vi "Convert EGU to V.vi"(0 "Sensors Info":T1(array[cluster])=[{"Sensor Name"="AI 0", "Sensor Info"={"Manufacturer"="", "Model"="", "Serial Number"=""}, "Last Cal Info"={"Last Calibration Date"=3153588337.646, "Calibrator"="", "Cal Duration"=0}, "Voltage Range"={"High Limit"=5.0, "Low Limit"=-5.0}, "EGU Range"={"High Limit"=-10000.0, "Low Limit"=10000.0}, "Units"="ue", "Calibration Type"=enum."Calibrate Analog", "EGU List"=[0.0, 10000.0, 20000.0], "Voltage List"=[0.0, 5.0, 7.0], "Coefficients"=[5.90433951730418e-12, -142.85714285714278, 428.5714285714284], "Order"=2, "Algorithm"=enum."SVD", "Max Error % of Full Scale"=0.0, "Max Mean Squared Error"=0.0, "Use Error %"=FALSE, "Use MSE"=FALSE, "Allow Manual Entry"=FALSE, "Max Stability Error"=2.0, "Max Error % of Reading"=0.0, "Use Error % of Reading"=FALSE}, {"Sensor Name"="AI 1", "Sensor Info"={"Manufacturer"="", "Model"="", "Serial Number"=""}, "Last Cal Info"={"Last Calibration Date"=3153957180.311, "Calibrator"="", "Cal Duration"=0}, "Voltage Range"={"High Limit"=5.0, "Low Limit"=-5.0}, "EGU Range"={"High Limit"=-10000.0, "Low Limit"=10000.0}, "Units"="ue", "Calibration Type"=enum."Calibrate Analog", "EGU List"=[0.0, 10000.0], "Voltage List"=[0.0, 5.0], "Coefficients"=[-0.0, 2000.0], "Order"=2, "Algorithm"=enum."SVD", "Max Error % of Full Scale"=0.0, "Max Mean Squared Error"=0.0, "Use Error %"=FALSE, "Use MSE"=FALSE, "Allow Manual Entry"=FALSE, "Max Stability Error"=2.0, "Max Error % of Reading"=0.0, "Use Error % of Reading"=FALSE}, {"Sensor Name"="AI 12", "Sensor Info"={"Manufacturer"="", "Model"="", "Serial Number"=""}, "Last Cal Info"={"Last Calibration Date"=3153952477.529, "Calibrator"="", "Cal Duration"=0}, "Voltage Range"={"High Limit"=0.0, "Low Limit"=10.0}, "EGU Range"={"High Limit"=0.0, "Low Limit"=10.0}, "Units"="Volts", "Calibration Type"=enum."Calibrate Analog", "EGU List"=[0.0, 10000.0], "Voltage List"=[0.0, 5.0], "Coefficients"=[-0.0, 2000.0], "Order"=2, "Algorithm"=enum."SVD", "Max Error % of Full Scale"=0.0, "Max Mean Squared Error"=0.0, "Use Error %"=FALSE, "Use MSE"=FALSE, "Allow Manual Entry"=FALSE, "Max Stability Error"=2.0, "Max Error % of Reading"=0.0, "Use Error % of Reading"=FALSE}, {"Sensor Name"="AI 13", "Sensor Info"={"Manufacturer"="", "Model"="", "Serial Number"=""}, "Last Cal Info"={"Last Calibration Date"=3153952479.4309998, "Calibrator"="", "Cal Duration"=0}, "Voltage Range"={"High Limit"=0.0, "Low Limit"=10.0}, "EGU Range"={"High Limit"=0.0, "Low Limit"=10.0}, "Units"="Volts", "Calibration Type"=enum."Calibrate Analog", "EGU List"=[0.0, 10000.0], "Voltage List"=[0.0, 5.0], "Coefficients"=[-0.0, 2000.0], "Order"=2, "Algorithm"=enum."SVD", "Max Error % of Full Scale"=0.0, "Max Mean Squared Error"=0.0, "Use Error %"=FALSE, "Use MSE"=FALSE, "Allow Manual Entry"=FALSE, "Max Stability Error"=2.0, "Max Error % of Reading"=0.0, "Use Error % of Reading"=FALSE}, {"Sensor Name"="AI 14", "Sensor Info"={"Manufacturer"="", "Model"="", "Serial Number"=""}, "Last Cal Info"={"Last Calibration Date"=3153952481.104, "Calibrator"="", "Cal Duration"=0}, "Voltage Range"={"High Limit"=0.0, "Low Limit"=10.0}, "EGU Range"={"High Limit"=0.0, "Low Limit"=10.0}, "Units"="Volts", "Calibration Type"=enum."Calibrate Analog", "EGU List"=[0.0, 10000.0], "Voltage List"=[0.0, 5.0], "Coefficients"=[-0.0, 2000.0], "Order"=2, "Algorithm"=enum."SVD", "Max Error % of Full Scale"=0.0, "Max Mean Squared Error"=0.0, "Use Error %"=FALSE, "Use MSE"=FALSE, "Allow Manual Entry"=FALSE, "Max Stability Error"=2.0, "Max Error % of Reading"=0.0, "Use Error % of Reading"=FALSE}, {"Sensor Name"="AI 15", "Sensor Info"={"Manufacturer"="", "Model"="", "Serial Number"=""}, "Last Cal Info"={"Last Calibration Date"=3153952482.786, "Calibrator"="", "Cal Duration"=0}, "Voltage Range"={"High Limit"=0.0, "Low Limit"=10.0}, "EGU Range"={"High Limit"=0.0, "Low Limit"=10.0}, "Units"="Volts", "Calibration Type"=enum."Calibrate Analog", "EGU List"=[0.0, 10000.0], "Voltage List"=[0.0, 5.0], "Coefficients"=[-0.0, 2000.0], "Order"=2, "Algorithm"=enum."SVD", "Max Error % of Full Scale"=0.0, "Max Mean Squared Error"=0.0, "Use Error %"=FALSE, "Use MSE"=FALSE, "Allow Manual Entry"=FALSE, "Max Stability Error"=2.0, "Max Error % of Reading"=0.0, "Use Error % of Reading"=FALSE}, {"Sensor Name"="AI 2", "Sensor Info"={"Manufacturer"="", "Model"="", "Serial Number"=""}, "Last Cal Info"={"Last Calibration Date"=3153588342.192, "Calibrator"="", "Cal Duration"=0}, "Voltage Range"={"High Limit"=5.0, "Low Limit"=-5.0}, "EGU Range"={"High Limit"=-10000.0, "Low Limit"=10000.0}, "Units"="ue", "Calibration Type"=enum."Calibrate Analog", "EGU List"=[0.0, 10000.0], "Voltage List"=[0.0, 5.0], "Coefficients"=[-0.0, 2000.0], "Order"=2, "Algorithm"=enum."SVD", "Max Error % of Full Scale"=0.0, "Max Mean Squared Error"=0.0, "Use Error %"=FALSE, "Use MSE"=FALSE, "Allow Manual Entry"=FALSE, "Max Stability Error"=2.0, "Max Error % of Reading"=0.0, "Use Error % of Reading"=FALSE}, {"Sensor Name"="AI 2", "Sensor Info"={"Manufacturer"="", "Model"="", "Serial Number"=""}, "Last Cal Info"={"Last Calibration Date"=3153844419.694, "Calibrator"="", "Cal Duration"=0}, "Voltage Range"={"High Limit"=0.0, "Low Limit"=10.0}, "EGU Range"={"High Limit"=0.0, "Low Limit"=10.0}, "Units"="Volts", "Calibration Type"=enum."Calibrate Analog", "EGU List"=[0.0, 10000.0], "Voltage List"=[0.0, 5.0], "Coefficients"=[-0.0, 2000.0], "Order"=2, "Algorithm"=enum."SVD", "Max Error % of Full Scale"=0.0, "Max Mean Squared Error"=0.0, "Use Error %"=FALSE, "Use MSE"=FALSE, "Allow Manual Entry"=FALSE, "Max Stability Error"=2.0, "Max Error % of Reading"=0.0, "Use Error % of Reading"=FALSE}, {"Sensor Name"="AI 3", "Sensor Info"={"Manufacturer"="", "Model"="", "Serial Number"=""}, "Last Cal Info"={"Last Calibration Date"=3153588411.1809998, "Calibrator"="", "Cal Duration"=0}, "Voltage Range"={"High Limit"=5.0, "Low Limit"=-5.0}, "EGU Range"={"High Limit"=-10000.0, "Low Limit"=10000.0}, "Units"="ue", "Calibration Type"=enum."Calibrate Analog", "EGU List"=[0.0, 10.0], "Voltage List"=[0.0, 5.0], "Coefficients"=[-0.0, 2.0], "Order"=2, "Algorithm"=enum."SVD", "Max Error % of Full Scale"=0.0, "Max Mean Squared Error"=0.0, "Use Error %"=FALSE, "Use MSE"=FALSE, "Allow Manual Entry"=FALSE, "Max Stability Error"=2.0, "Max Error % of Reading"=0.0, "Use Error % of Reading"=FALSE}, {"Sensor Name"="AI 3", "Sensor Info"={"Manufacturer"="", "Model"="", "Serial Number"=""}, "Last Cal Info"={"Last Calibration Date"=3153952458.0099998, "Calibrator"="", "Cal Duration"=0}, "Voltage Range"={"High Limit"=0.0, "Low Limit"=10.0}, "EGU Range"={"High Limit"=0.0, "Low Limit"=10.0}, "Units"="Volts", "Calibration Type"=enum."Calibrate Analog", "EGU List"=[0.0, 10000.0], "Voltage List"=[0.0, 5.0], "Coefficients"=[-0.0, 2000.0], "Order"=2, "Algorithm"=enum."SVD", "Max Error % of Full Scale"=0.0, "Max Mean Squared Error"=0.0, "Use Error %"=FALSE, "Use MSE"=FALSE, "Allow Manual Entry"=FALSE, "Max Stability Error"=2.0, "Max Error % of Reading"=0.0, "Use Error % of Reading"=FALSE}, {"Sensor Name"="AI 4", "Sensor Info"={"Manufacturer"="", "Model"="", "Serial Number"=""}, "Last Cal Info"={"Last Calibration Date"=3153952461.015, "Calibrator"="", "Cal Duration"=0}, "Voltage Range"={"High Limit"=0.0, "Low Limit"=10.0}, "EGU Range"={"High Limit"=0.0, "Low Limit"=10.0}, "Units"="Volts", "Calibration Type"=enum."Calibrate Analog", "EGU List"=[0.0, 10000.0], "Voltage List"=[0.0, 5.0], "Coefficients"=[-0.0, 2000.0], "Order"=2, "Algorithm"=enum."SVD", "Max Error % of Full Scale"=0.0, "Max Mean Squared Error"=0.0, "Use Error %"=FALSE, "Use MSE"=FALSE, "Allow Manual Entry"=FALSE, "Max Stability Error"=2.0, "Max Error % of Reading"=0.0, "Use Error % of Reading"=FALSE}, {"Sensor Name"="AI 5", "Sensor Info"={"Manufacturer"="", "Model"="", "Serial Number"=""}, "Last Cal Info"={"Last Calibration Date"=3153952462.988, "Calibrator"="", "Cal Duration"=0}, "Voltage Range"={"High Limit"=0.0, "Low Limit"=10.0}, "EGU Range"={"High Limit"=0.0, "Low Limit"=10.0}, "Units"="Volts", "Calibration Type"=enum."Calibrate Analog", "EGU List"=[0.0, 10000.0], "Voltage List"=[0.0, 5.0], "Coefficients"=[-0.0, 2000.0], "Order"=2, "Algorithm"=enum."SVD", "Max Error % of Full Scale"=0.0, "Max Mean Squared Error"=0.0, "Use Error %"=FALSE, "Use MSE"=FALSE, "Allow Manual Entry"=FALSE, "Max Stability Error"=2.0, "Max Error % of Reading"=0.0, "Use Error % of Reading"=FALSE}, {"Sensor Name"="AI 6", "Sensor Info"={"Manufacturer"="", "Model"="", "Serial Number"=""}, "Last Cal Info"={"Last Calibration Date"=3153952464.56, "Calibrator"="", "Cal Duration"=0}, "Voltage Range"={"High Limit"=0.0, "Low Limit"=10.0}, "EGU Range"={"High Limit"=0.0, "Low Limit"=10.0}, "Units"="Volts", "Calibration Type"=enum."Calibrate Analog", "EGU List"=[0.0, 10000.0], "Voltage List"=[0.0, 5.0], "Coefficients"=[-0.0, 2000.0], "Order"=2, "Algorithm"=enum."SVD", "Max Error % of Full Scale"=0.0, "Max Mean Squared Error"=0.0, "Use Error %"=FALSE, "Use MSE"=FALSE, "Allow Manual Entry"=FALSE, "Max Stability Error"=2.0, "Max Error % of Reading"=0.0, "Use Error % of Reading"=FALSE}, {"Sensor Name"="AI 7", "Sensor Info"={"Manufacturer"="", "Model"="", "Serial Number"=""}, "Last Cal Info"={"Last Calibration Date"=3153952466.733, "Calibrator"="", "Cal Duration"=0}, "Voltage Range"={"High Limit"=0.0, "Low Limit"=10.0}, "EGU Range"={"High Limit"=0.0, "Low Limit"=10.0}, "Units"="Volts", "Calibration Type"=enum."Calibrate Analog", "EGU List"=[0.0, 10000.0], "Voltage List"=[0.0, 5.0], "Coefficients"=[-0.0, 2000.0], "Order"=2, "Algorithm"=enum."SVD", "Max Error % of Full Scale"=0.0, "Max Mean Squared Error"=0.0, "Use Error %"=FALSE, "Use MSE"=FALSE, "Allow Manual Entry"=FALSE, "Max Stability Error"=2.0, "Max Error % of Reading"=0.0, "Use Error % of Reading"=FALSE}, {"Sensor Name"="AI 8", "Sensor Info"={"Manufacturer"="", "Model"="", "Serial Number"=""}, "Last Cal Info"={"Last Calibration Date"=3153952468.716, "Calibrator"="", "Cal Duration"=0}, "Voltage Range"={"High Limit"=0.0, "Low Limit"=10.0}, "EGU Range"={"High Limit"=0.0, "Low Limit"=10.0}, "Units"="Volts", "Calibration Type"=enum."Calibrate Analog", "EGU List"=[0.0, 10000.0], "Voltage List"=[0.0, 5.0], "Coefficients"=[-0.0, 2000.0], "Order"=2, "Algorithm"=enum."SVD", "Max Error % of Full Scale"=0.0, "Max Mean Squared Error"=0.0, "Use Error %"=FALSE, "Use MSE"=FALSE, "Allow Manual Entry"=FALSE, "Max Stability Error"=2.0, "Max Error % of Reading"=0.0, "Use Error % of Reading"=FALSE}, {"Sensor Name"="AI 9", "Sensor Info"={"Manufacturer"="", "Model"="", "Serial Number"=""}, "Last Cal Info"={"Last Calibration Date"=3153952470.388, "Calibrator"="", "Cal Duration"=0}, "Voltage Range"={"High Limit"=0.0, "Low Limit"=10.0}, "EGU Range"={"High Limit"=0.0, "Low Limit"=10.0}, "Units"="Volts", "Calibration Type"=enum."Calibrate Analog", "EGU List"=[0.0, 10000.0], "Voltage List"=[0.0, 5.0], "Coefficients"=[-0.0, 2000.0], "Order"=2, "Algorithm"=enum."SVD", "Max Error % of Full Scale"=0.0, "Max Mean Squared Error"=0.0, "Use Error %"=FALSE, "Use MSE"=FALSE, "Allow Manual Entry"=FALSE, "Max Stability Error"=2.0, "Max Error % of Reading"=0.0, "Use Error % of Reading"=FALSE}, {"Sensor Name"="Scott", "Sensor Info"={"Manufacturer"="", "Model"="", "Serial Number"=""}, "Last Cal Info"={"Last Calibration Date"=0.0, "Calibrator"="", "Cal Duration"=0}, "Voltage Range"={"High Limit"=10.0, "Low Limit"=-10.0}, "EGU Range"={"High Limit"=10.0, "Low Limit"=-10.0}, "Units"="Volts", "Calibration Type"=enum."Calibrate Analog", "EGU List"=[0.0, 10.0, 20.0], "Voltage List"=[0.0, 10.0, 20.0], "Coefficients"=[3.116871181724906e-15, 0.9999999999999998], "Order"=1, "Algorithm"=enum."SVD", "Max Error % of Full Scale"=0.0, "Max Mean Squared Error"=0.0, "Use Error %"=FALSE, "Use MSE"=FALSE, "Allow Manual Entry"=FALSE, "Max Stability Error"=2.0, "Max Error % of Reading"=0.0, "Use Error % of Reading"=FALSE}, {"Sensor Name"="Strain 0", "Sensor Info"={"Manufacturer"="", "Model"="", "Serial Number"=""}, "Last Cal Info"={"Last Calibration Date"=3153137126.758, "Calibrator"="", "Cal Duration"=0}, "Voltage Range"={"High Limit"=5.0, "Low Limit"=-5.0}, "EGU Range"={"High Limit"=-10000.0, "Low Limit"=10000.0}, "Units"="ue", "Calibration Type"=enum."Calibrate Analog", "EGU List"=[0.0, 10000.0], "Voltage List"=[0.0, 5.0], "Coefficients"=[3.658184866139891e-14, 1999.9999999999998], "Order"=1, "Algorithm"=enum."SVD", "Max Error % of Full Scale"=0.0, "Max Mean Squared Error"=0.0, "Use Error %"=FALSE, "Use MSE"=FALSE, "Allow Manual Entry"=FALSE, "Max Stability Error"=2.0, "Max Error % of Reading"=0.0, "Use Error % of Reading"=FALSE}, {"Sensor Name"="Strain 1", "Sensor Info"={"Manufacturer"="", "Model"="", "Serial Number"=""}, "Last Cal Info"={"Last Calibration Date"=3153957185.548, "Calibrator"="", "Cal Duration"=0}, "Voltage Range"={"High Limit"=5.0, "Low Limit"=-5.0}, "EGU Range"={"High Limit"=-10000.0, "Low Limit"=10000.0}, "Units"="ue", "Calibration Type"=enum."Calibrate Analog", "EGU List"=[0.0, 10000.0], "Voltage List"=[0.0, 5.0], "Coefficients"=[-0.0, 2000.0], "Order"=2, "Algorithm"=enum."SVD", "Max Error % of Full Scale"=0.0, "Max Mean Squared Error"=0.0, "Use Error %"=FALSE, "Use MSE"=FALSE, "Allow Manual Entry"=FALSE, "Max Stability Error"=2.0, "Max Error % of Reading"=0.0, "Use Error % of Reading"=FALSE}, {"Sensor Name"="Strain 10", "Sensor Info"={"Manufacturer"="", "Model"="", "Serial Number"=""}, "Last Cal Info"={"Last Calibration Date"=3153138160.091, "Calibrator"="", "Cal Duration"=0}, "Voltage Range"={"High Limit"=5.0, "Low Limit"=-5.0}, "EGU Range"={"High Limit"=-10000.0, "Low Limit"=10000.0}, "Units"="ue", "Calibration Type"=enum."Calibrate Analog", "EGU List"=[0.0, 10000.0], "Voltage List"=[0.0, 5.0], "Coefficients"=[3.658184866139891e-14, 1999.9999999999998], "Order"=1, "Algorithm"=enum."SVD", "Max Error % of Full Scale"=0.0, "Max Mean Squared Error"=0.0, "Use Error %"=FALSE, "Use MSE"=FALSE, "Allow Manual Entry"=FALSE, "Max Stability Error"=2.0, "Max Error % of Reading"=0.0, "Use Error % of Reading"=FALSE}, {"Sensor Name"="Strain 11", "Sensor Info"={"Manufacturer"="", "Model"="", "Serial Number"=""}, "Last Cal Info"={"Last Calibration Date"=3153138164.5379996, "Calibrator"="", "Cal Duration"=0}, "Voltage Range"={"High Limit"=5.0, "Low Limit"=-5.0}, "EGU Range"={"High Limit"=-10000.0, "Low Limit"=10000.0}, "Units"="ue", "Calibration Type"=enum."Calibrate Analog", "EGU List"=[0.0, 10000.0], "Voltage List"=[0.0, 5.0], "Coefficients"=[3.658184866139891e-14, 1999.9999999999998], "Order"=1, "Algorithm"=enum."SVD", "Max Error % of Full Scale"=0.0, "Max Mean Squared Error"=0.0, "Use Error %"=FALSE, "Use MSE"=FALSE, "Allow Manual Entry"=FALSE, "Max Stability Error"=2.0, "Max Error % of Reading"=0.0, "Use Error % of Reading"=FALSE}, {"Sensor Name"="Strain 12", "Sensor Info"={"Manufacturer"="", "Model"="", "Serial Number"=""}, "Last Cal Info"={"Last Calibration Date"=3153138186.1689997, "Calibrator"="", "Cal Duration"=0}, "Voltage Range"={"High Limit"=5.0, "Low Limit"=-5.0}, "EGU Range"={"High Limit"=-10000.0, "Low Limit"=10000.0}, "Units"="ue", "Calibration Type"=enum."Calibrate Analog", "EGU List"=[0.0, 10000.0], "Voltage List"=[0.0, 5.0], "Coefficients"=[3.658184866139891e-14, 1999.9999999999998], "Order"=1, "Algorithm"=enum."SVD", "Max Error % of Full Scale"=0.0, "Max Mean Squared Error"=0.0, "Use Error %"=FALSE, "Use MSE"=FALSE, "Allow Manual Entry"=FALSE, "Max Stability Error"=2.0, "Max Error % of Reading"=0.0, "Use Error % of Reading"=FALSE}, {"Sensor Name"="Strain 13", "Sensor Info"={"Manufacturer"="", "Model"="", "Serial Number"=""}, "Last Cal Info"={"Last Calibration Date"=3153138190.555, "Calibrator"="", "Cal Duration"=0}, "Voltage Range"={"High Limit"=5.0, "Low Limit"=-5.0}, "EGU Range"={"High Limit"=-10000.0, "Low Limit"=10000.0}, "Units"="ue", "Calibration Type"=enum."Calibrate Analog", "EGU List"=[0.0, 10000.0], "Voltage List"=[0.0, 5.0], "Coefficients"=[3.658184866139891e-14, 1999.9999999999998], "Order"=1, "Algorithm"=enum."SVD", "Max Error % of Full Scale"=0.0, "Max Mean Squared Error"=0.0, "Use Error %"=FALSE, "Use MSE"=FALSE, "Allow Manual Entry"=FALSE, "Max Stability Error"=2.0, "Max Error % of Reading"=0.0, "Use Error % of Reading"=FALSE}, {"Sensor Name"="Strain 14", "Sensor Info"={"Manufacturer"="", "Model"="", "Serial Number"=""}, "Last Cal Info"={"Last Calibration Date"=3153138195.632, "Calibrator"="", "Cal Duration"=0}, "Voltage Range"={"High Limit"=5.0, "Low Limit"=-5.0}, "EGU Range"={"High Limit"=-10000.0, "Low Limit"=10000.0}, "Units"="ue", "Calibration Type"=enum."Calibrate Analog", "EGU List"=[0.0, 10000.0], "Voltage List"=[0.0, 5.0], "Coefficients"=[3.658184866139891e-14, 1999.9999999999998], "Order"=1, "Algorithm"=enum."SVD", "Max Error % of Full Scale"=0.0, "Max Mean Squared Error"=0.0, "Use Error %"=FALSE, "Use MSE"=FALSE, "Allow Manual Entry"=FALSE, "Max Stability Error"=2.0, "Max Error % of Reading"=0.0, "Use Error % of Reading"=FALSE}, {"Sensor Name"="Strain 15", "Sensor Info"={"Manufacturer"="", "Model"="", "Serial Number"=""}, "Last Cal Info"={"Last Calibration Date"=3153138198.4059997, "Calibrator"="", "Cal Duration"=0}, "Voltage Range"={"High Limit"=5.0, "Low Limit"=-5.0}, "EGU Range"={"High Limit"=-10000.0, "Low Limit"=10000.0}, "Units"="ue", "Calibration Type"=enum."Calibrate Analog", "EGU List"=[0.0, 10000.0], "Voltage List"=[0.0, 5.0], "Coefficients"=[3.658184866139891e-14, 1999.9999999999998], "Order"=1, "Algorithm"=enum."SVD", "Max Error % of Full Scale"=0.0, "Max Mean Squared Error"=0.0, "Use Error %"=FALSE, "Use MSE"=FALSE, "Allow Manual Entry"=FALSE, "Max Stability Error"=2.0, "Max Error % of Reading"=0.0, "Use Error % of Reading"=FALSE}, {"Sensor Name"="Strain 2", "Sensor Info"={"Manufacturer"="", "Model"="", "Serial Number"=""}, "Last Cal Info"={"Last Calibration Date"=3153138100.5759997, "Calibrator"="", "Cal Duration"=0}, "Voltage Range"={"High Limit"=5.0, "Low Limit"=-5.0}, "EGU Range"={"High Limit"=-10000.0, "Low Limit"=10000.0}, "Units"="ue", "Calibration Type"=enum."Calibrate Analog", "EGU List"=[0.0, 10000.0], "Voltage List"=[0.0, 5.0], "Coefficients"=[3.658184866139891e-14, 1999.9999999999998], "Order"=1, "Algorithm"=enum."SVD", "Max Error % of Full Scale"=0.0, "Max Mean Squared Error"=0.0, "Use Error %"=FALSE, "Use MSE"=FALSE, "Allow Manual Entry"=FALSE, "Max Stability Error"=2.0, "Max Error % of Reading"=0.0, "Use Error % of Reading"=FALSE}, {"Sensor Name"="Strain 3", "Sensor Info"={"Manufacturer"="", "Model"="", "Serial Number"=""}, "Last Cal Info"={"Last Calibration Date"=3153138104.2419996, "Calibrator"="", "Cal Duration"=0}, "Voltage Range"={"High Limit"=5.0, "Low Limit"=-5.0}, "EGU Range"={"High Limit"=-10000.0, "Low Limit"=10000.0}, "Units"="ue", "Calibration Type"=enum."Calibrate Analog", "EGU List"=[0.0, 10000.0], "Voltage List"=[0.0, 5.0], "Coefficients"=[3.658184866139891e-14, 1999.9999999999998], "Order"=1, "Algorithm"=enum."SVD", "Max Error % of Full Scale"=0.0, "Max Mean Squared Error"=0.0, "Use Error %"=FALSE, "Use MSE"=FALSE, "Allow Manual Entry"=FALSE, "Max Stability Error"=2.0, "Max Error % of Reading"=0.0, "Use Error % of Reading"=FALSE}, {"Sensor Name"="Strain 4", "Sensor Info"={"Manufacturer"="", "Model"="", "Serial Number"=""}, "Last Cal Info"={"Last Calibration Date"=3153138108.4979997, "Calibrator"="", "Cal Duration"=0}, "Voltage Range"={"High Limit"=5.0, "Low Limit"=-5.0}, "EGU Range"={"High Limit"=-10000.0, "Low Limit"=10000.0}, "Units"="ue", "Calibration Type"=enum."Calibrate Analog", "EGU List"=[0.0, 10000.0], "Voltage List"=[0.0, 5.0], "Coefficients"=[3.658184866139891e-14, 1999.9999999999998], "Order"=1, "Algorithm"=enum."SVD", "Max Error % of Full Scale"=0.0, "Max Mean Squared Error"=0.0, "Use Error %"=FALSE, "Use MSE"=FALSE, "Allow Manual Entry"=FALSE, "Max Stability Error"=2.0, "Max Error % of Reading"=0.0, "Use Error % of Reading"=FALSE}, {"Sensor Name"="Strain 5", "Sensor Info"={"Manufacturer"="", "Model"="", "Serial Number"=""}, "Last Cal Info"={"Last Calibration Date"=3153138145.2799997, "Calibrator"="", "Cal Duration"=0}, "Voltage Range"={"High Limit"=5.0, "Low Limit"=-5.0}, "EGU Range"={"High Limit"=-10000.0, "Low Limit"=10000.0}, "Units"="ue", "Calibration Type"=enum."Calibrate Analog", "EGU List"=[0.0, 10000.0], "Voltage List"=[0.0, 5.0], "Coefficients"=[3.658184866139891e-14, 1999.9999999999998], "Order"=1, "Algorithm"=enum."SVD", "Max Error % of Full Scale"=0.0, "Max Mean Squared Error"=0.0, "Use Error %"=FALSE, "Use MSE"=FALSE, "Allow Manual Entry"=FALSE, "Max Stability Error"=2.0, "Max Error % of Reading"=0.0, "Use Error % of Reading"=FALSE}, {"Sensor Name"="Strain 6", "Sensor Info"={"Manufacturer"="", "Model"="", "Serial Number"=""}, "Last Cal Info"={"Last Calibration Date"=3153138148.725, "Calibrator"="", "Cal Duration"=0}, "Voltage Range"={"High Limit"=5.0, "Low Limit"=-5.0}, "EGU Range"={"High Limit"=-10000.0, "Low Limit"=10000.0}, "Units"="ue", "Calibration Type"=enum."Calibrate Analog", "EGU List"=[0.0, 10000.0], "Voltage List"=[0.0, 5.0], "Coefficients"=[3.658184866139891e-14, 1999.9999999999998], "Order"=1, "Algorithm"=enum."SVD", "Max Error % of Full Scale"=0.0, "Max Mean Squared Error"=0.0, "Use Error %"=FALSE, "Use MSE"=FALSE, "Allow Manual Entry"=FALSE, "Max Stability Error"=2.0, "Max Error % of Reading"=0.0, "Use Error % of Reading"=FALSE}, {"Sensor Name"="Strain 7", "Sensor Info"={"Manufacturer"="", "Model"="", "Serial Number"=""}, "Last Cal Info"={"Last Calibration Date"=3153138151.539, "Calibrator"="", "Cal Duration"=0}, "Voltage Range"={"High Limit"=5.0, "Low Limit"=-5.0}, "EGU Range"={"High Limit"=-10000.0, "Low Limit"=10000.0}, "Units"="ue", "Calibration Type"=enum."Calibrate Analog", "EGU List"=[0.0, 10000.0], "Voltage List"=[0.0, 5.0], "Coefficients"=[3.658184866139891e-14, 1999.9999999999998], "Order"=1, "Algorithm"=enum."SVD", "Max Error % of Full Scale"=0.0, "Max Mean Squared Error"=0.0, "Use Error %"=FALSE, "Use MSE"=FALSE, "Allow Manual Entry"=FALSE, "Max Stability Error"=2.0, "Max Error % of Reading"=0.0, "Use Error % of Reading"=FALSE}, {"Sensor Name"="Strain 8", "Sensor Info"={"Manufacturer"="", "Model"="", "Serial Number"=""}, "Last Cal Info"={"Last Calibration Date"=3153138154.273, "Calibrator"="", "Cal Duration"=0}, "Voltage Range"={"High Limit"=5.0, "Low Limit"=-5.0}, "EGU Range"={"High Limit"=-10000.0, "Low Limit"=10000.0}, "Units"="ue", "Calibration Type"=enum."Calibrate Analog", "EGU List"=[0.0, 10000.0], "Voltage List"=[0.0, 5.0], "Coefficients"=[3.658184866139891e-14, 1999.9999999999998], "Order"=1, "Algorithm"=enum."SVD", "Max Error % of Full Scale"=0.0, "Max Mean Squared Error"=0.0, "Use Error %"=FALSE, "Use MSE"=FALSE, "Allow Manual Entry"=FALSE, "Max Stability Error"=2.0, "Max Error % of Reading"=0.0, "Use Error % of Reading"=FALSE}, {"Sensor Name"="Strain 9", "Sensor Info"={"Manufacturer"="", "Model"="", "Serial Number"=""}, "Last Cal Info"={"Last Calibration Date"=3153138157.3469996, "Calibrator"="", "Cal Duration"=0}, "Voltage Range"={"High Limit"=5.0, "Low Limit"=-5.0}, "EGU Range"={"High Limit"=-10000.0, "Low Limit"=10000.0}, "Units"="ue", "Calibration Type"=enum."Calibrate Analog", "EGU List"=[0.0, 10000.0], "Voltage List"=[0.0, 5.0], "Coefficients"=[3.658184866139891e-14, 1999.9999999999998], "Order"=1, "Algorithm"=enum."SVD", "Max Error % of Full Scale"=0.0, "Max Mean Squared Error"=0.0, "Use Error %"=FALSE, "Use MSE"=FALSE, "Allow Manual Entry"=FALSE, "Max Stability Error"=2.0, "Max Error % of Reading"=0.0, "Use Error % of Reading"=FALSE}], 5 "Config":T2={"DAQ Settings"={"Trigger Type"=enum."Timed", "Trigger Samples"=1000, "Pretrigger Samples"=0, "Trigger Interval"=1.0, "Time Units"=FALSE, "Auto Save"=FALSE, "Sample Rate"=2.0, "Select Analog"=FALSE, "Trigger Value"=0.0, "Trigger Stop Method"=enum."Use Samples Value to Stop Trigger", "Rate Sec/Min"=FALSE, "Save Mode"=enum."Single File", "File Size Limit"=0.0, "Log File Type"=enum."Basic", "Trigger Data Index"=0}, "Channels"=[], "Header"={"TA Number"="WTI", "Test Name"="TEST", "Serial Number"="12345", "Technician"="Comments"}, "Graph Settings"={"Graph Labels"=[], [], [], [], [], [], [], [], [], [], [], [], [], "Graph Toggles"=[], "Axis Toggles"=[], "Graph Range"=enum."1"}, "Test Limits"=[], "All Type Info"=[], "Save Mode"=enum."Single File"} {"DAQ Settings"."Trigger Interval" min=0.0; "DAQ Settings"."Pretrigger Samples" min=0; "DAQ Settings"."Trigger Samples" min=0}, 7 "Channel Name":string, 9 "EGU Value":dbl) -> (8 "Channel ID":string, 10 "Voltage":dbl)   [LabVIEW 2019]
uses:
  Type Defs and Controls/Sensor Config.ctl
  Type Defs and Controls/DAQ Settings.ctl
  Type Defs and Controls/Trigger Stop Method.ctl
  Type Defs and Controls/Log File Type.ctl
  Type Defs and Controls/Channel Config.ctl
  Type Defs and Controls/Header.ctl
  Type Defs and Controls/Graph Settings Type Def.ctl
  Type Defs and Controls/Test Limits.ctl
  Type Defs and Controls/All Part Info.ctl
  Type Defs and Controls/Part Info.ctl
  <vilib>/Analysis/NI_AALBase.lvlib
  <vilib>/Analysis/NI_AALPro.lvlib
panel:
  # "EGU"
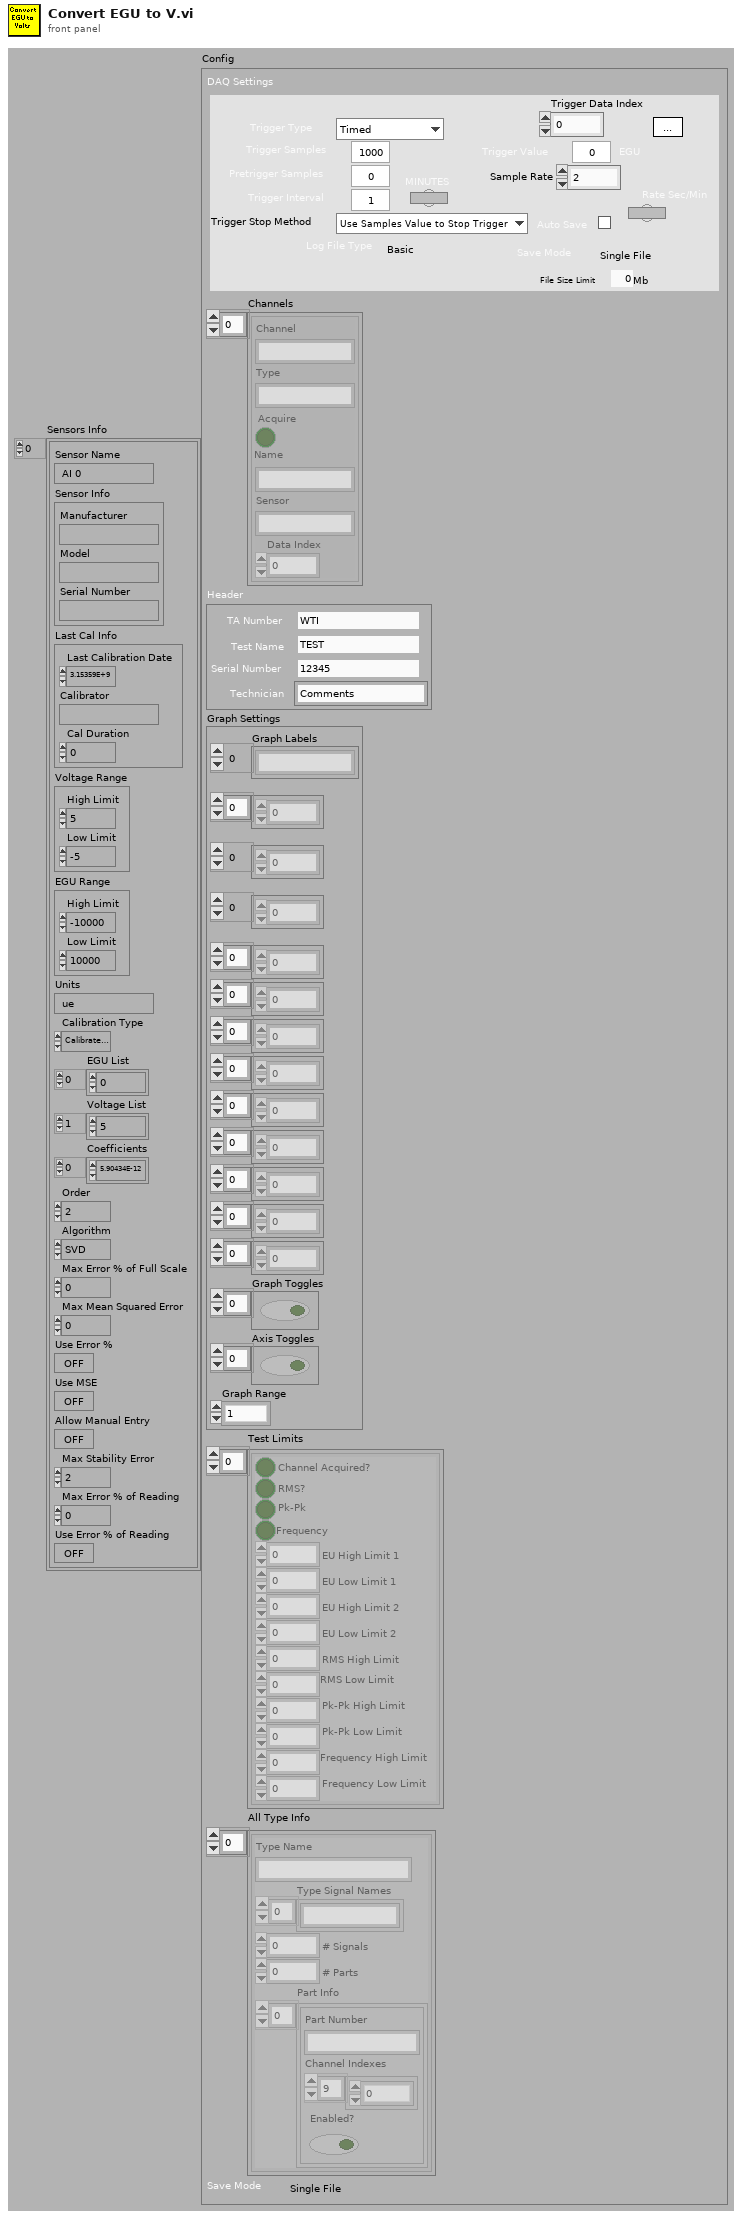
[diagram p1: front panel]
types:
  T1 = cluster{"Sensor Name":string, "Sensor Info":cluster{"Manufacturer":string, "Model":string, "Serial Number":string}, "Last Cal Info":cluster{"Last Calibration Date":dbl, "Calibrator":string, "Cal Duration":i32}, "Voltage Range":cluster{"High Limit":dbl, "Low Limit":dbl}, "EGU Range":cluster{"High Limit":dbl, "Low Limit":dbl}, "Units":string, "Calibration Type":enum16{"Calibrate Analog", "Compare Analog Calibration"}, "EGU List":dbl[], "Voltage List":dbl[], "Coefficients":dbl[], "Order":i32, "Algorithm":enum32{"SVD", "Givens", "Givens2", "Householder", "LU Decomposition", "Cholesky"}, "Max Error % of Full Scale":dbl, "Max Mean Squared Error":dbl, "Use Error %":bool, "Use MSE":bool, "Allow Manual Entry":bool, "Max Stability Error":dbl, "Max Error % of Reading":dbl, "Use Error % of Reading":bool}[]
  T2 = typedef "Sensor Config.ctl" = cluster{"DAQ Settings":T3, "Channels":T6[], "Header":T7, "Graph Settings":T8, "Test Limits":T9[], "All Type Info":T10, "Save Mode":enum16{"Single File", "Segmented Files", "New File at Midnight"}}
  T3 = typedef "DAQ Settings.ctl" = cluster{"Trigger Type":enum16{"Manual", "Timed", "Analog Rising", "Analog Falling"}, "Trigger Samples":i32, "Pretrigger Samples":i32, "Trigger Interval":dbl, "Time Units":bool, "Auto Save":bool, "Sample Rate":dbl, "Select Analog":bool, "Trigger Value":dbl, "Trigger Stop Method":T4, "Rate Sec/Min":bool, "Save Mode":enum16{"Single File", "Segmented Files", "New File at Midnight"}, "File Size Limit":dbl, "Log File Type":T5, "Trigger Data Index":u32}
  T4 = typedef "Trigger Stop Method.ctl" = enum16{"Use Samples Value to Stop Trigger", "Use Threshold to Stop Trigger"}
  T5 = typedef "Log File Type.ctl" = enum16{"Basic", "RTS"}
  T6 = typedef "Channel Config.ctl" = cluster{"Channel":string, "Type":string, "Acquire":bool, "Name":string, "Sensor":string, "Data Index":u32}
  T7 = typedef "Header.ctl" = cluster{"TA Number":string, "Test Name":string, "Serial Number":string, "Technician":string}
  T8 = typedef "Graph Settings Type Def.ctl" = cluster{"Graph Labels":string[], u8[], i16[], u32[], u8[], u8[], u8[], u32[], u8[], u8[], u8[], dbl[], dbl[], "Graph Toggles":bool[], "Axis Toggles":bool[], "Graph Range":enum16{"1", "2", "3", "4", "5", "10", "15", "30", "60"}}
  T9 = typedef "Test Limits.ctl" = cluster{"Channel Acquired?":bool, "RMS?":bool, "Pk-Pk":bool, "Frequency":bool, "EU High Limit 1":dbl, "EU Low Limit 1":dbl, "EU High Limit 2":dbl, "EU Low Limit 2":dbl, "RMS High Limit":dbl, "RMS Low Limit":dbl, "Pk-Pk High Limit ":dbl, "Pk-Pk Low Limit":dbl, "Frequency High Limit":dbl, "Frequency Low Limit":dbl}
  T10 = typedef "All Part Info.ctl" = cluster{"Type Name":string, "Type Signal Names":string[], "# Signals":i32, "# Parts":i32, "Part Info":T11[]}[]
  T11 = typedef "Part Info.ctl" = cluster{"Part Number":string, "Channel Indexes":u16[], "Enabled?":bool}
  T12 = cluster{"Sensor Name":string, "Sensor Info":cluster{"Manufacturer":string, "Model":string, "Serial Number":string}, "Last Cal Info":cluster{"Last Calibration Date":dbl, "Calibrator":string, "Cal Duration":i32}, "Voltage Range":cluster{"High Limit":dbl, "Low Limit":dbl}, "EGU Range":cluster{"High Limit":dbl, "Low Limit":dbl}, "Units":string, "Calibration Type":enum16{"Calibrate Analog", "Compare Analog Calibration"}, "EGU List":dbl[], "Voltage List":dbl[], "Coefficients":dbl[], "Order":i32, "Algorithm":enum32{"SVD", "Givens", "Givens2", "Householder", "LU Decomposition", "Cholesky"}, "Max Error % of Full Scale":dbl, "Max Mean Squared Error":dbl, "Use Error %":bool, "Use MSE":bool, "Allow Manual Entry":bool, "Max Stability Error":dbl, "Max Error % of Reading":dbl, "Use Error % of Reading":bool}
  T13 = enum32{"SVD", "Givens", "Givens2", "Householder", "LU Decomposition", "Cholesky"}
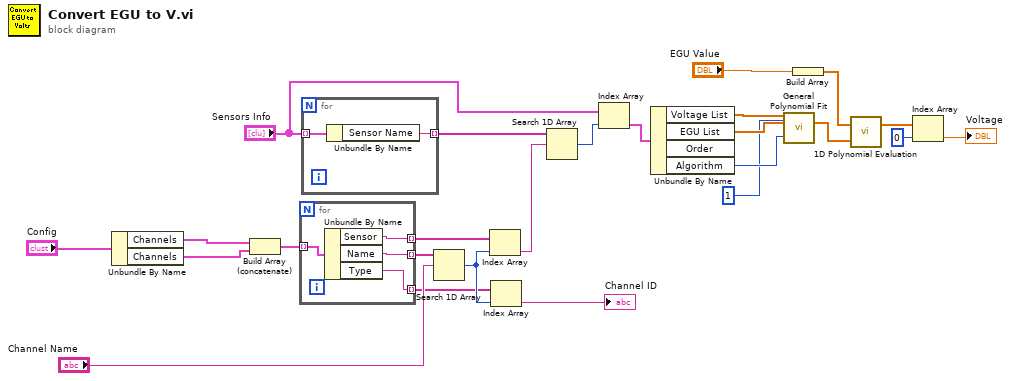
[diagram p0: block diagram]
diagram:
  n1 = Unbundle By Name("Config") -> ("Channels"=w24:T6[], "Channels"=w23:T6[])
  n2 = Build Array (concatenate)(w24, w23) -> (w22:T6[])
  n3 = for {
    tunnel: w22 -> [w29] mode=indexing
    tunnel: [w28] -> w21 mode=indexing
    tunnel: [w27] -> w20 mode=indexing
    tunnel: [w26] -> w3 mode=indexing
    n4 = Unbundle By Name(w29) -> ("Sensor"=w27:string, "Name"=w28:string, "Type"=w26:string)
  }
  n5 = for {
    tunnel: "Sensors Info" -> [w31] mode=indexing
    tunnel: [w30] -> w18 mode=indexing
    n6 = Unbundle By Name(w31) -> ("Sensor Name"=w30:string)
  }
  n7 = Search 1D Array(1D array=w21, element="Channel Name") -> (index of element=w4:i32)  [unwired: 1 in]
  n8 = Index Array(array=w20, index=w4) -> (element=w19:string)
  n9 = Index Array(array=w3, index=w4) -> (element=→"Channel ID":string)
  n10 = Search 1D Array(1D array=w18, element=w19) -> (index of element=w17:i32)  [unwired: 1 in]
  n11 = Index Array(array="Sensors Info", index=w17) -> (element=w15:T12)
  n12 = Unbundle By Name(w15) -> ("Voltage List"=w14:dbl[], "EGU List"=w13:dbl[], "Algorithm"=w7:T13)  [unwired: 1 out]
  n13 = call <vilib>:"General Polynomial Fit.vi"("Y"=w14, "polynomial order"=1, "X"=w13, "algorithm"=w7) -> ("Polynomial Coefficients"=w5:dbl[])  [unwired: 8 in, 3 out]
  n14 = Build Array("EGU Value") -> (w6:dbl[])
  n15 = call <vilib>:"1D Polynomial Evaluation.vi"("Coefficients: a"=w5, "X"=w6) -> ("Y"=w11:dbl[])  [unwired: 1 out]
  n16 = Index Array(array=w11, index=0) -> (element=→"Voltage":dbl)
